vi "parse_RxUDPmessageBuffer.vi"(10 "MsgRead(1)":u32=1, 11 "ReadBuffer":u8[](array[numeric])) -> (0 "error info":u32[](array[numeric]), 1 "msg size":u32[](array[numeric]), 2 "IrigTime":T1(array[cluster]), 3 "Message Data":u8[][](array[numeric]))   [LabVIEW 2020, in "AIM664LV.lvlib"]
uses:
  AIM664LV.lvlib
  bsp/AFDX_TargetIndependentAdmin/FdxFwIrig2StructIrigCvi.vi
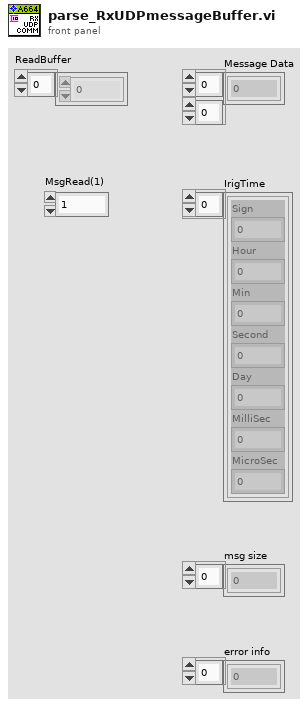
[diagram p1: front panel]
types:
  T1 = cluster{"Sign":i32, "Hour":u32, "Min":u32, "Second":u32, "Day":u32, "MilliSec":u32, "MicroSec":u32}[]
  T2 = cluster{"Sign":i32, "Hour":u32, "Min":u32, "Second":u32, "Day":u32, "MilliSec":u32, "MicroSec":u32}
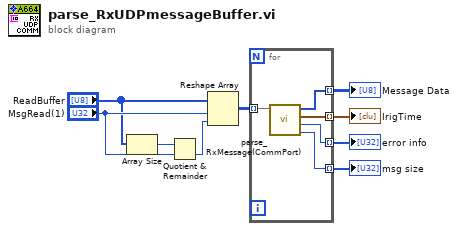
[diagram p0: block diagram]
diagram:
  n1 = Array Size(array="ReadBuffer") -> (size(s)=w8:i32)
  n2 = Quotient & Remainder(x=w8, y="MsgRead(1)") -> (floor(x/y)=w7:u32)  [unwired: 1 out]
  n3 = Reshape Array("ReadBuffer", "MsgRead(1)", w7) -> (w9:u8[][])
  n4 = for {
    tunnel: w9 -> [w14] mode=indexing
    tunnel: [w13] -> w6 mode=indexing
    tunnel: [w12] -> w5 mode=indexing
    tunnel: [w11] -> w4 mode=indexing
    tunnel: [w10] -> w3 mode=indexing
    n5 = call "parse_RxMessage(CommPort).vi"("ReadBuffer In"=w14) -> ("msg size"=w10:u32, "error info"=w11:u32, "IrigTime"=w12:T2, "Message Data"=w13:u8[])  [unwired: 7 in]
  }
  "Message Data" <- w6
  "IrigTime" <- w5
  "msg size" <- w3
  "error info" <- w4
